vi "LLSize.vi"(8 "error in (no error)":errorcluster, 11 "LinkedList in":refnum<class "LinkedList.lvclass">) -> (0 "error out":errorcluster, 2 "size":i32, 3 "LinkedList out":refnum<class "LinkedList.lvclass">)   [LabVIEW 2013, in "LinkedList.lvclass"]
doc: "Finds the size (how many nodes) of the linked list."
uses:
  LinkedList.lvclass
  LinkedList.lvclass/LinkedList.ctl
  LLNode/LLNode.lvclass
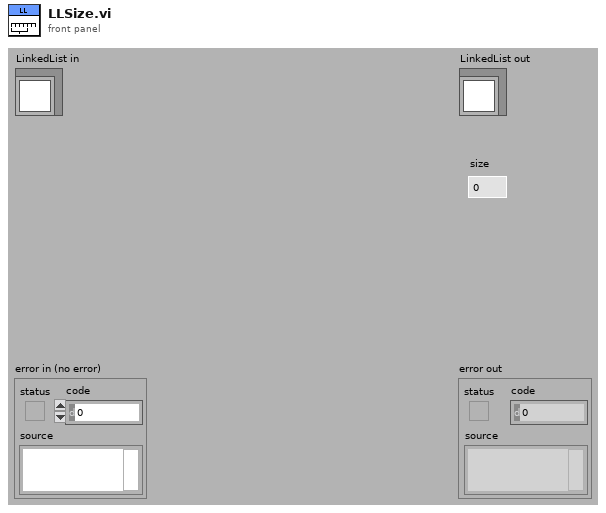
[diagram p1: front panel]
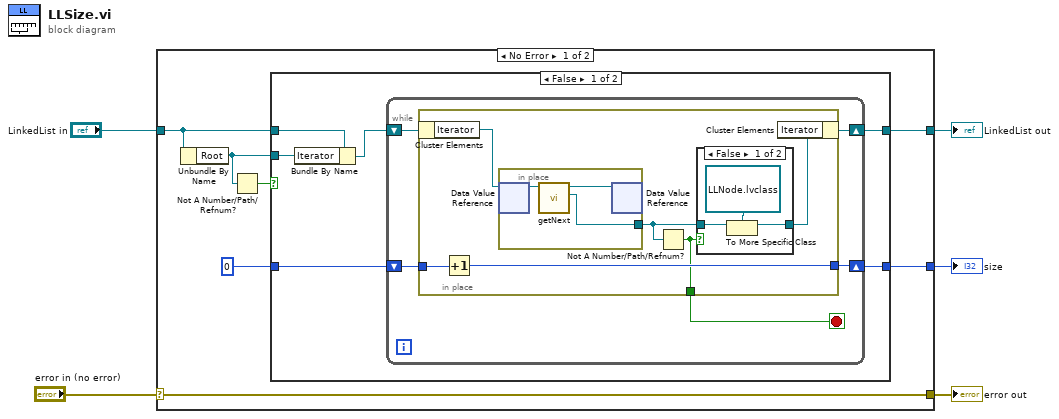
[diagram p0: block diagram]
diagram:
  n1 = case shown="No Error" "error in (no error)" {
    selector: "error in (no error)" -> [w12 w38]
    tunnel: [w12 w38] -> w4
    tunnel: [w9 w37] -> w2
    tunnel: "LinkedList in" -> [w11 w37]
    tunnel: [w8 _] -> w1
    frame No Error {
      n2 = Unbundle By Name(w11) -> ("Root"=w6:refnum<data-value>)
      n3 = Not A Number/Path/Refnum?(number/path/refnum=w6) -> (NaN/Path/Refnum?=w7:bool)
      n4 = case shown="False" w7 {
        tunnel: w6 -> [w18 _]
        tunnel: w11 -> [w17 w36]
        tunnel: 0 -> [w15 _]
        tunnel: [w14 w36] -> w9
        tunnel: [w13 _] -> w8
        frame False {
          n5 = Bundle By Name(cluster=w17, "Iterator"=w18) -> (w16:refnum<class "LinkedList.lvclass">)
          n6 = while {
            shift-right: [w20] -> w14
            shift-left: w16 -> [w23]
            shift-right: [w21] -> w13
            shift-left: w15 -> [w22]
            stop <- w19 stop-if-true
            n7 = in-place {
              in-place-border: w22 -> [w29]
              in-place-border: [w28] -> w21
              in-place-border: [w24] -> w19
              n8 = in-place-cluster #1(w23) -> ("Iterator"=w27:refnum<data-value>)
              n9 = Increment(x=w29) -> (x+1=w28:i32)
              n10 = in-place {
                in-place-border: [w33] -> w26
                n11 = in-place-dvr #2(w27) -> (w35:refnum<class "LLNode.lvclass">)  [unwired: 1 out]
                n12 = call "getNext.vi"("LLNode in"=w35) -> ("next"=w33:refnum<data-value>, "LLNode out"=w34:refnum<class "LLNode.lvclass">)  [unwired: 8 in, 1 out]
                n13 = in-place-dvr #2(w34) -> ()  [unwired: 2 out]
              }
              n14 = Not A Number/Path/Refnum?(number/path/refnum=w26) -> (NaN/Path/Refnum?=w24:bool)
              n15 = case shown="False" w24 {
                tunnel: w26 -> [w32 _]
                tunnel: [w30 _] -> w25
                frame False {
                  n16 = To More Specific Class(target class=refnum<data-value> refnum ("Root"), reference=w32) -> (specific class reference=w30:refnum<data-value>)  [unwired: 1 in, 1 out]
                }
                frame True {
                }
              }
              n17 = in-place-cluster #1("Iterator"=w25) -> (w20:refnum<class "LinkedList.lvclass">)
            }
          }
        }
        frame True {
        }
      }
    }
    frame Error {
    }
  }
  "error out" <- w4
  "LinkedList out" <- w2
  "size" <- w1
